vi "current monitor3.vi"() -> ()   [LabVIEW 2010]
uses:
  <vilib>/Utility/file.llb/Write To Spreadsheet File (DBL).vi
  <userlib>/Nanonis Prog Interface V5/Nanonis Prog Interface.lvlib
panel:
  in  "Start":bool
  in  "Loop delay":dbl
  in  "Convert to nm/s?":bool caption="Spectrum Analyzer 2"
  out "Spectrum Analyzer 2":cluster{"f0":dbl, "df":dbl, "values":dbl[]}(graph)
  in  "Spectrum Analyzer2":bool caption="Spectrum Analyzer 2"
  out "error out":errorcluster
  in  "Path":path
  out "Spectrum Analyzer":cluster{"f0":dbl, "df":dbl, "values":dbl[]}(graph)
  out "Current (A)":sgl format="%#_6p"
  out "Current":cluster{"Current (A)":dbl, dbl}[](graph)
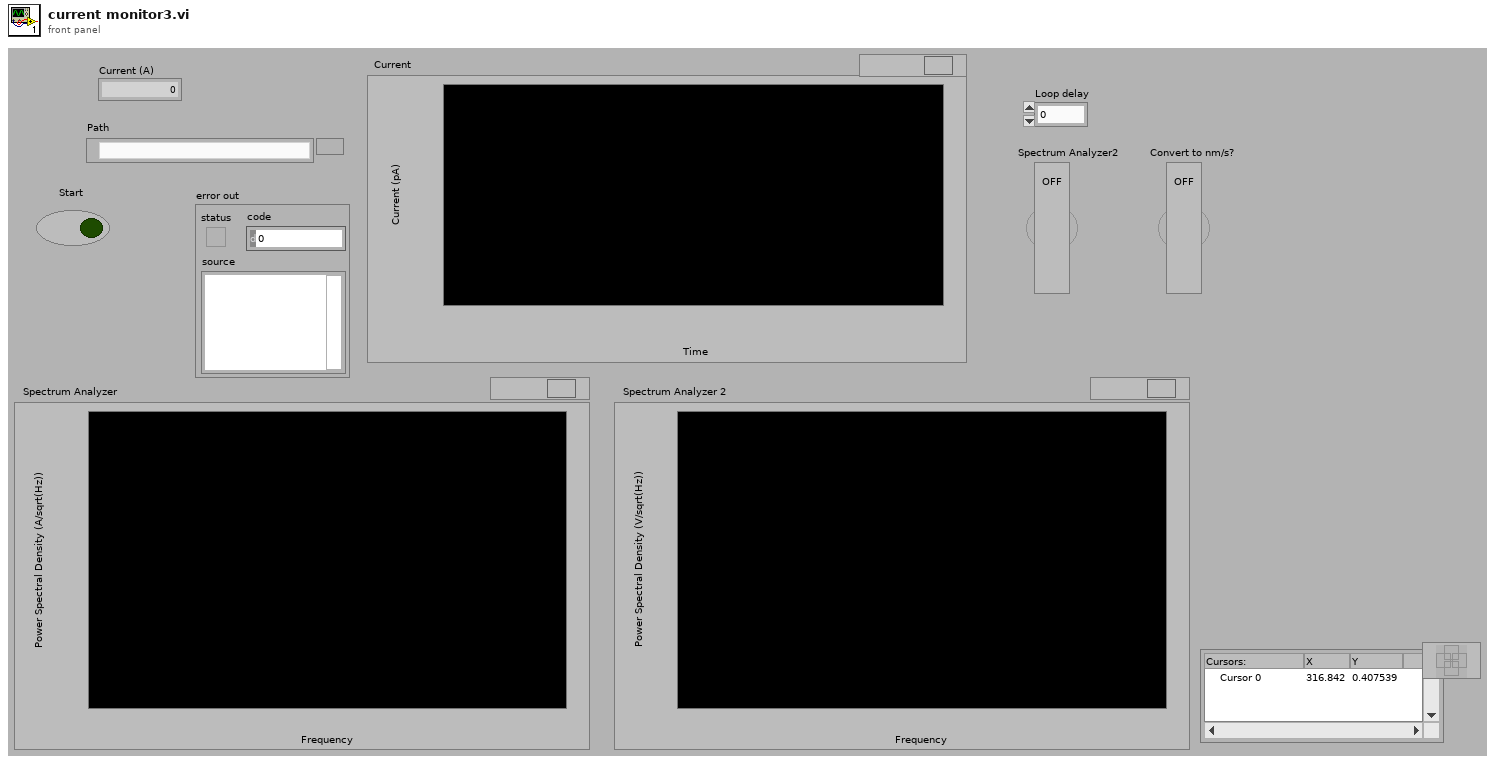
[diagram p1: front panel]
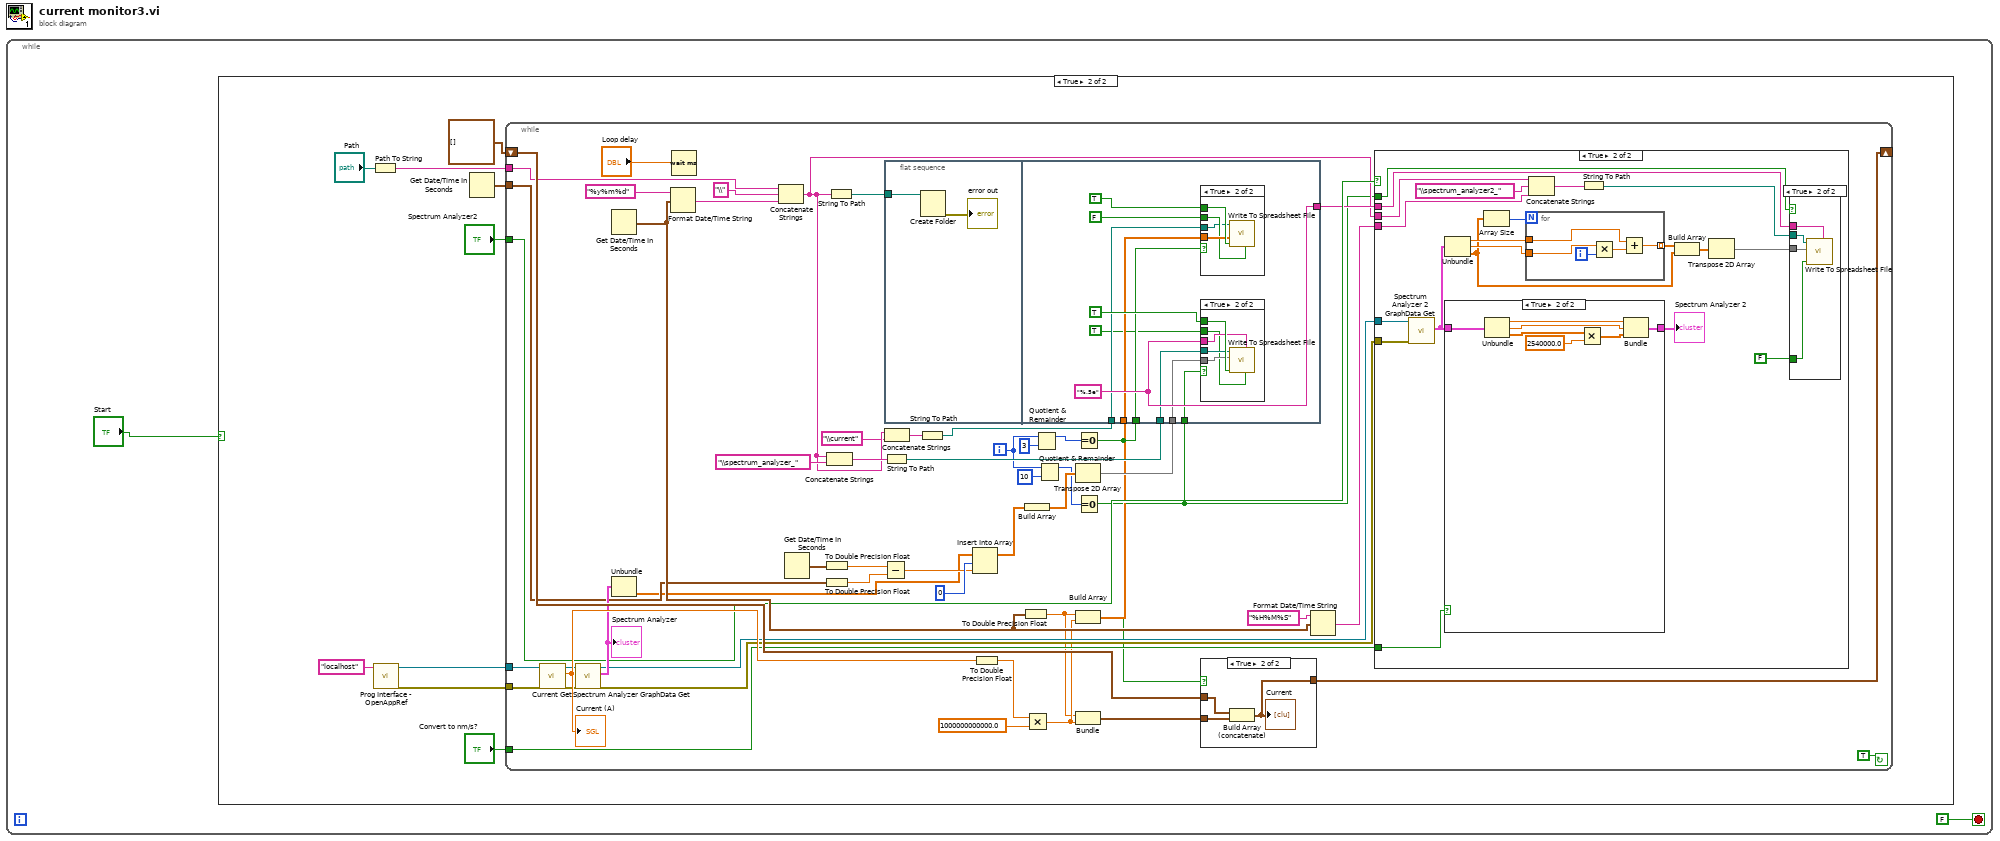
[diagram p0: block diagram]
diagram:
  n1 = while {
    stop <- FALSE stop-if-true
    n2 = case shown="True" "Start" {
      frame False {
      }
      frame True {
        n3 = Path To String(path="Path") -> (string=w6:string)
        n4 = call <userlib>:"Prog Interface - OpenAppRef.vi"("Machine name (local machine IP)"="localhost" ("machine name (localhost)")) -> ("Error out"=w10:errorcluster, "Application reference"=w11:refnum<vi>)  [unwired: 5 in]
        n5 = Get Date/Time In Seconds() -> (seconds since 1Jan1904=w3:timestamp)
        n6 = while {
          tunnel: w11 -> [w63]
          tunnel: w10 -> [w62]
          shift-right: [w59] -> _
          shift-left: cluster{dbl, dbl}[] [] -> [w60]
          tunnel: w6 -> [w48]
          tunnel: "Spectrum Analyzer2" -> [w38]
          tunnel: "Convert to nm/s?" -> [w36]
          tunnel: w3 -> [w14]
          i -> [w23]
          stop <- TRUE continue-if-true
          n7 = call <userlib>:"Current Get.vi"("Error in (no error)"=w62, "Application ref in"=w63) -> ("Error out"=w54:errorcluster, "Current (A)"=w58:sgl, "Application ref out"=w55:refnum<vi>)  [unwired: 5 in]
          "Current (A)" <- w58
          n8 = call <userlib>:"Spectrum Analyzer GraphData Get.vi"("Error in (no error)"=w54, "Application ref in"=w55) -> ("Error out"=w39:errorcluster, "FFT data"=w53:cluster{"f0":dbl, "df":dbl, "values":dbl[]}, "Application ref out"=w40:refnum<vi>)  [unwired: 7 in]
          "Spectrum Analyzer" <- w53
          n9 = Get Date/Time In Seconds() -> (seconds since 1Jan1904=w49:timestamp)
          n10 = Unbundle(w53) -> ("values"=w13:dbl[])  [unwired: 2 out]
          n11 = Format Date/Time String(time format string (%c)="%y%m%d", seconds (now)=w49) -> (date/time string=w46:string)  [unwired: 1 in]
          n12 = Wait (ms)(milliseconds to wait="Loop delay") -> ()  [unwired: 1 out]
          n13 = Concatenate Strings(w48, "\\" ("string"), w46) -> (w34:string)
          n14 = Get Date/Time In Seconds() -> (seconds since 1Jan1904=w17:timestamp)
          n15 = To Double Precision Float(number=w17) -> (double precision float=w16:dbl)
          n16 = To Double Precision Float(number=w14) -> (double precision float=w15:dbl)
          n17 = Concatenate Strings(w34, "\\spectrum_analyzer_" ("string")) -> (w43:string)
          n18 = String To Path(string=w34) -> (path=w47:path)
          n19 = Subtract(x=w16, y=w15) -> (x-y=w18:dbl)
          n20 = String To Path(string=w43) -> (path=w51:path)
          n21 = flat-sequence {
            tunnel: w47 -> [w107]
            tunnel: w51 -> [w111]
            tunnel: w41 -> [w112]
            tunnel: [w117] -> w37
            tunnel: w35 -> [w115]
            tunnel: w31 -> [w113]
            tunnel: w26 -> [w110]
            tunnel: w22 -> [w109]
            frame #0 {
              n22 = Create Folder(path (use dialog)=w107) -> (error out=→"error out":errorcluster)  [unwired: 2 in, 2 out]
            }
            frame #1 {
              w117 = "%.5e" ("format (%.3f)")
              n23 = case shown="True" w109 {
                tunnel: TRUE ("append to file? (new file:F)") -> [_ w122]
                tunnel: w115 -> [_ w121]
                tunnel: FALSE ("transpose? (no:F)") -> [_ w120]
                tunnel: w113 -> [_ w119]
                frame False {
                }
                frame True {
                  n24 = call-poly <vilib>:"Write To Spreadsheet File.vi"("transpose? (no:F)"=w120, "append to file? (new file:F)"=w122, "1D data"=w121, "file path (dialog if empty)"=w119) -> ()  [unwired: 4 in, 1 out]
                }
              }
              n25 = case shown="True" w110 {
                tunnel: TRUE ("append to file? (new file:F)") -> [_ w127]
                tunnel: w117 -> [_ w126]
                tunnel: w112 -> [_ w125]
                tunnel: w111 -> [_ w124]
                tunnel: TRUE -> [_ w123]
                frame False {
                }
                frame True {
                  n26 = call-poly <vilib>:"Write To Spreadsheet File.vi"("transpose? (no:F)"=w123, "format (%.3f)"=w126, "append to file? (new file:F)"=w127, "2D data"=w125, "file path (dialog if empty)"=w124) -> ()  [unwired: 3 in, 1 out]
                }
              }
            }
          }
          n27 = Concatenate Strings(w34, "\\current" ("string")) -> (w32:string)
          n28 = String To Path(string=w32) -> (path=w31:path)
          n29 = Insert Into Array(array=w13, index=0, new element=w18) -> (w19:dbl[])
          n30 = To Double Precision Float(number=w58) -> (double precision float=w57:dbl)
          n31 = To Double Precision Float(number=w49) -> (double precision float=w29:dbl)
          n32 = Build Array(w19) -> (w42:dbl[][])
          n33 = Multiply(x=w57, y=1000000000000.0) -> (x*y=w30:dbl)
          n34 = Quotient & Remainder(x=w23, y=3) -> (x-y*floor(x/y)=w24:i32)  [unwired: 1 out]
          n35 = Quotient & Remainder(x=w23, y=10) -> (x-y*floor(x/y)=w27:i32)  [unwired: 1 out]
          n36 = Transpose 2D Array(2D array=w42) -> (transposed array=w41:dbl[][])
          n37 = Build Array(w29, w30) -> (w35:dbl[])
          n38 = Bundle(w29, w30) -> (w61:cluster{dbl, dbl})  [unwired: 1 in]
          n39 = Equal To 0?(x=w24) -> (x = 0?=w22:bool)
          n40 = Equal To 0?(x=w27) -> (x = 0?=w26:bool)
          n41 = case shown="True" w22 {
            tunnel: w61 -> [_ w68]
            tunnel: w60 -> [w65 w67]
            tunnel: [w65 w66] -> w59
            frame False {
            }
            frame True {
              n42 = Build Array (concatenate)(w67, w68) -> (w66:cluster{dbl, dbl}[])
              "Current" <- w66
            }
          }
          n43 = Format Date/Time String(time format string (%c)="%H%M%S", seconds (now)=w49) -> (date/time string=w21:string)  [unwired: 1 in]
          n44 = case shown="True" w38 {
            tunnel: w40 -> [_ w88]
            tunnel: w39 -> [_ w87]
            tunnel: w34 -> [_ w78]
            tunnel: w21 -> [_ w77]
            tunnel: w37 -> [_ w73]
            tunnel: w36 -> [_ w70]
            tunnel: w26 -> [_ w69]
            frame False {
            }
            frame True {
              n45 = call <userlib>:"Spectrum Analyzer 2 GraphData Get.vi"("Error in (no error)"=w87, "Application ref in"=w88) -> ("FFT data"=w72:cluster{"f0":dbl, "df":dbl, "values":dbl[]})  [unwired: 7 in, 2 out]
              n46 = Unbundle(w72) -> ("f0"=w85:dbl, "df"=w84:dbl, "values"=w82:dbl[])
              n47 = case shown="True" w70 {
                tunnel: w72 -> [w93 w100]
                tunnel: [w93 w99] -> w71
                frame False {
                }
                frame True {
                  n48 = Unbundle(w100) -> ("f0"=w98:dbl, "df"=w97:dbl, "values"=w96:dbl[])
                  n49 = Multiply(x=w96, y=2540000.0) -> (x*y=w95:dbl[])
                  n50 = Bundle("f0"=w98, "df"=w97, w95) -> (w99:cluster{"f0":dbl, "df":dbl, dbl[]})  [unwired: 1 in]
                }
              }
              "Spectrum Analyzer 2" <- w71
              n51 = Array Size(array=w82) -> (size(s)=w86:i32)
              n52 = for {
                N: w86 -> [_]
                tunnel: w85 -> [w105]
                tunnel: w84 -> [w102]
                tunnel: [w101] -> w81 mode=indexing
                i -> [w103]
                n53 = Multiply(x=w102, y=w103) -> (x*y=w104:dbl)
                n54 = Add(x=w105, y=w104) -> (x+y=w101:dbl)
              }
              n55 = Concatenate Strings(w78, "\\spectrum_analyzer2_" ("string"), w77) -> (w74:string)
              n56 = String To Path(string=w74) -> (path=w75:path)
              n57 = Build Array(w81, w82) -> (w83:dbl[][])
              n58 = Transpose 2D Array(2D array=w83) -> (transposed array=w79:dbl[][])
              n59 = case shown="True" w69 {
                tunnel: FALSE ("append to file? (new file:F)") -> [_ w92]
                tunnel: w79 -> [_ w91]
                tunnel: w75 -> [_ w90]
                tunnel: w73 -> [_ w89]
                frame False {
                }
                frame True {
                  n60 = call-poly <vilib>:"Write To Spreadsheet File.vi"("format (%.3f)"=w89, "append to file? (new file:F)"=w92, "2D data"=w91, "file path (dialog if empty)"=w90) -> ()  [unwired: 4 in, 1 out]
                }
              }
            }
          }
        }
      }
    }
  }
